vi "5.vi"() -> ()   [LabVIEW 2017]
panel:
  out "波形图":dbl[][](graph)
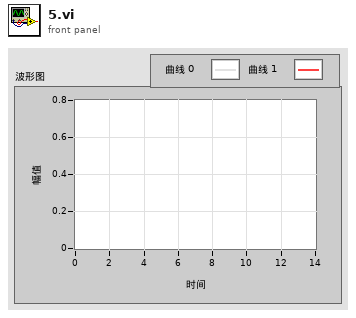
[diagram p1: front panel]
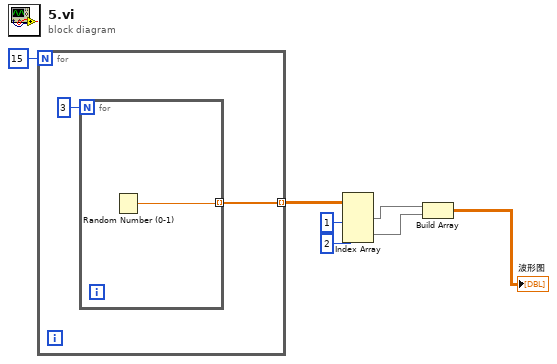
[diagram p0: block diagram]
diagram:
  n1 = for {
    N: 15 -> [_]
    tunnel: [w8] -> w6 mode=indexing
    n2 = for {
      N: 3 -> [_]
      tunnel: [w10] -> w8 mode=indexing
      n3 = Random Number (0-1)() -> (number: 0 to 1=w10:dbl)
    }
  }
  n4 = Index Array(array=w6, index (col) #1=1 ("禁用的索引 (列)"), index (col) #2=2 ("索引 (列)")) -> (element #1=w3:dbl[], element #2=w2:dbl[])  [unwired: 2 in]
  n5 = Build Array(w3, w2) -> (→"波形图":dbl[][])
